vi "U2PCoeff.vi"(2 "Numeric":dbl, 3 "Kappa00":dbl[](array[numeric]), 4 "RB000":dbl[](array[numeric])) -> (0 "Array":dbl[](array[numeric]), 1 "Array 2":dbl[](array[numeric]))   [LabVIEW 2014]
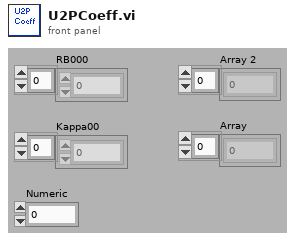
[diagram p1: front panel]
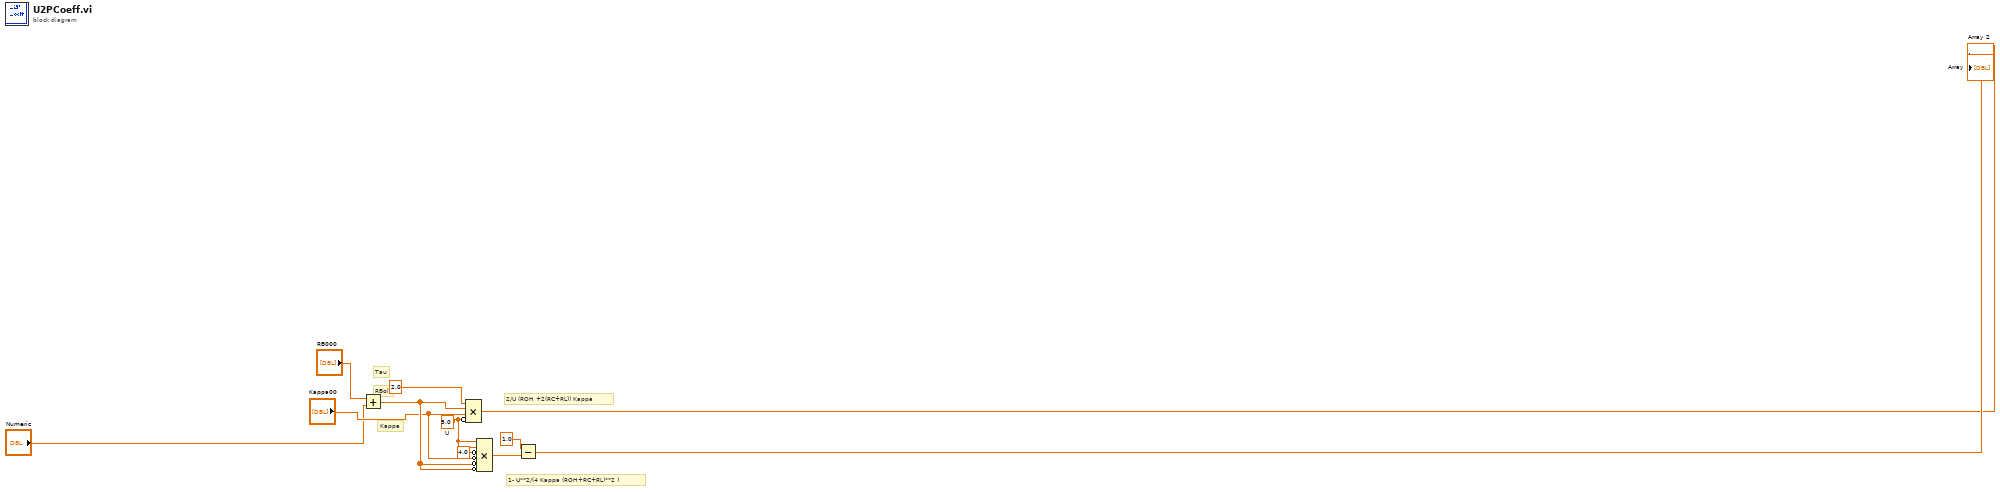
[diagram p0: block diagram]
diagram:
  w3 = 5.0  # U
  # "1- U**2/(4 Kappa (ROH+RC+RL)**2 )"
  # "2/U (ROH +2(RC+RL)) Kappa"
  # "Kappa"
  # "RBol"
  # "Tau"
  n1 = Add(x="RB000", y="Numeric") -> (x+y=w11:dbl[])
  n2 = Compound Arithmetic op=MULTIPLY(2.0, w11, "Kappa00", invert w3) -> (→"Array 2":dbl[])
  n3 = Compound Arithmetic op=MULTIPLY(w3, w3, invert 4.0 ("value"), invert "Kappa00", invert w11, invert w11) -> (w6:dbl[])
  n4 = Subtract(x=1.0, y=w6) -> (x-y=→"Array":dbl[])
